vi "FlatToRichgrpc_reflection_v1alpha_ServerReflectionResponse.vi"(5 "OutputClusterType":T1, 11 "InputCluster":T3) -> (3 "OutputCluster":T1)   [LabVIEW 2025, in "reflection_server.lvlib"]
uses:
  reflection_server.lvlib
  grpc_reflection_v1alpha_ServerReflectionResponse_Flat.ctl
  grpc_reflection_v1alpha_ServerReflectionRequest_Flat.ctl
  grpc_reflection_v1alpha_ExtensionRequest_Flat.ctl
  grpc_reflection_v1alpha_FileDescriptorResponse_Flat.ctl
  grpc_reflection_v1alpha_ExtensionNumberResponse_Flat.ctl
  grpc_reflection_v1alpha_ListServiceResponse_Flat.ctl
  grpc_reflection_v1alpha_ServiceResponse_Flat.ctl
  grpc_reflection_v1alpha_ErrorResponse_Flat.ctl
  grpc_reflection_v1alpha_ServerReflectionResponse.ctl
  grpc_reflection_v1alpha_ServerReflectionRequest_message_request/grpc_reflection_v1alpha_ServerReflectionRequest_message_request.lvclass
  grpc_reflection_v1alpha_ServerReflectionResponse_message_response/grpc_reflection_v1alpha_ServerReflectionResponse_message_response.lvclass
  grpc_reflection_v1alpha_ServerReflectionRequest.ctl
  grpc_reflection_v1alpha_ServerReflectionRequest_message_request/grpc_reflection_v1alpha_ServerReflectionRequest_message_request.lvclass/grpc_reflection_v1alpha_ServerReflectionRequest_message_request.ctl
  grpc_reflection_v1alpha_ServerReflectionResponse_message_response/grpc_reflection_v1alpha_ServerReflectionResponse_message_response.lvclass/grpc_reflection_v1alpha_ServerReflectionResponse_message_response.ctl
  grpc_reflection_v1alpha_ServerReflectionRequest_message_request/Setfile_by_filename.vi
  grpc_reflection_v1alpha_ServerReflectionRequest_message_request/Setfile_containing_symbol.vi
  grpc_reflection_v1alpha_ServerReflectionRequest_message_request/Setfile_containing_extension.vi
  FlatToRichgrpc_reflection_v1alpha_ExtensionRequest.vi
  grpc_reflection_v1alpha_ServerReflectionRequest_message_request/Setall_extension_numbers_of_type.vi
  grpc_reflection_v1alpha_ServerReflectionRequest_message_request/Setlist_services.vi
  FlatToRichgrpc_reflection_v1alpha_ServiceResponse.vi
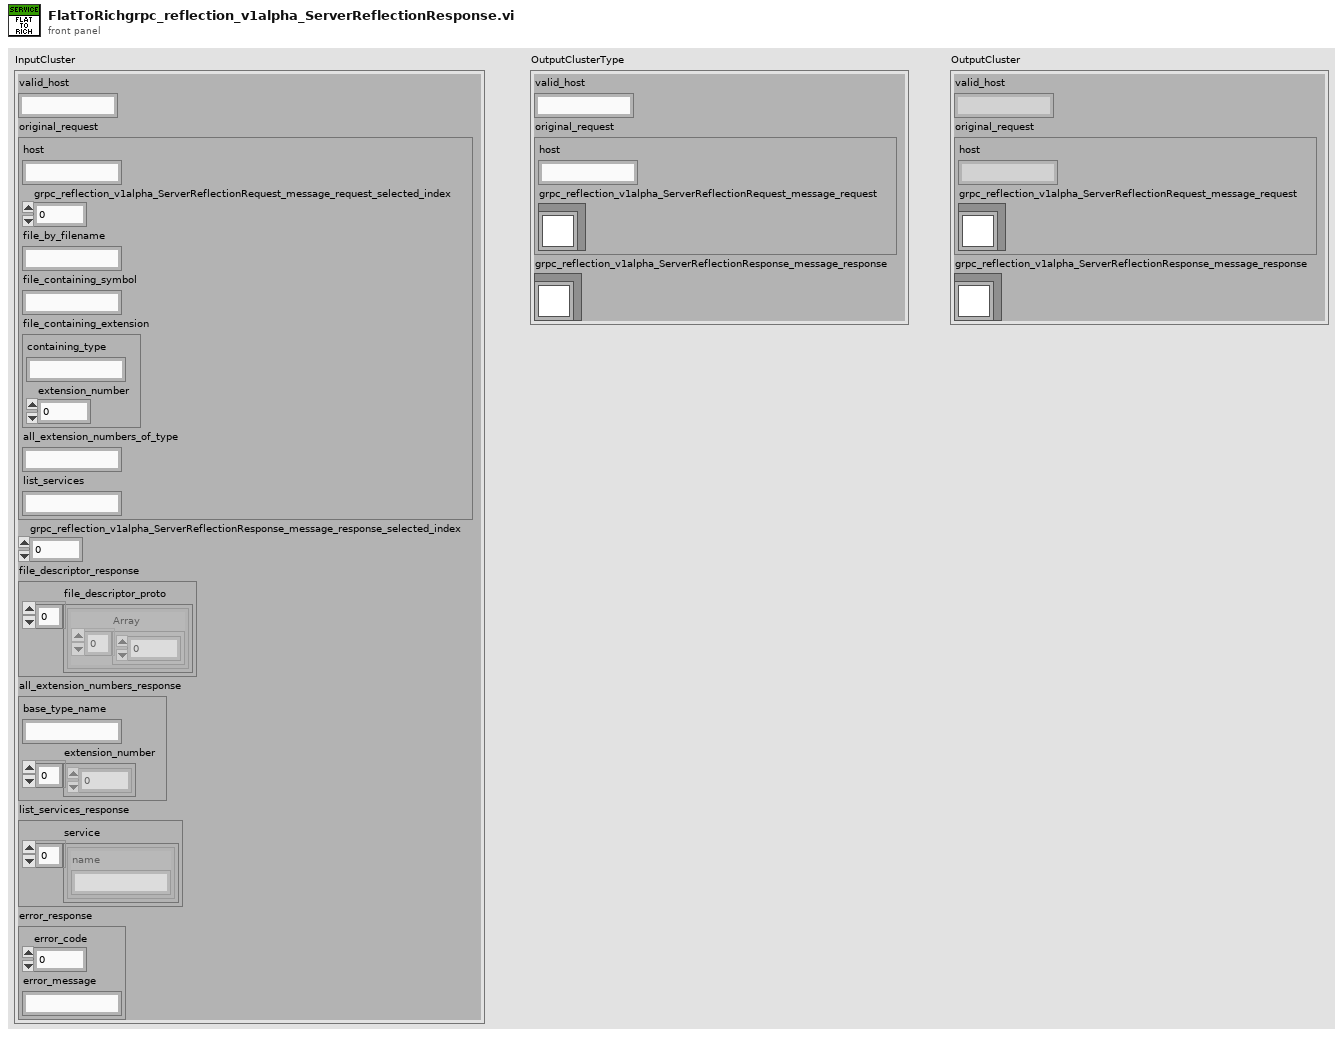
[diagram p1: front panel]
types:
  T1 = typedef "reflection_server.lvlib/grpc_reflection_v1alpha_ServerReflectionResponse.ctl" = cluster{"valid_host":string, "original_request":T2, "grpc_reflection_v1alpha_ServerReflectionResponse_message_response":refnum<class "grpc_reflection_v1alpha_ServerReflectionResponse_message_response.lvclass">}
  T2 = typedef "reflection_server.lvlib/grpc_reflection_v1alpha_ServerReflectionRequest.ctl" = cluster{"host":string, "grpc_reflection_v1alpha_ServerReflectionRequest_message_request":refnum<class "grpc_reflection_v1alpha_ServerReflectionRequest_message_request.lvclass">}
  T3 = typedef "reflection_server.lvlib/grpc_reflection_v1alpha_ServerReflectionResponse_Flat.ctl" = cluster{"valid_host":string, "original_request":T4, "grpc_reflection_v1alpha_ServerReflectionResponse_message_response_selected_index":i32, "file_descriptor_response":T6, "all_extension_numbers_response":T7, "list_services_response":T8, "error_response":T10}
  T4 = typedef "reflection_server.lvlib/grpc_reflection_v1alpha_ServerReflectionRequest_Flat.ctl" = cluster{"host":string, "grpc_reflection_v1alpha_ServerReflectionRequest_message_request_selected_index":i32, "file_by_filename":string, "file_containing_symbol":string, "file_containing_extension":T5, "all_extension_numbers_of_type":string, "list_services":string}
  T5 = typedef "reflection_server.lvlib/grpc_reflection_v1alpha_ExtensionRequest_Flat.ctl" = cluster{"containing_type":string, "extension_number":i32}
  T6 = typedef "reflection_server.lvlib/grpc_reflection_v1alpha_FileDescriptorResponse_Flat.ctl" = cluster{"file_descriptor_proto":cluster{"Array":u8[]}[]}
  T7 = typedef "reflection_server.lvlib/grpc_reflection_v1alpha_ExtensionNumberResponse_Flat.ctl" = cluster{"base_type_name":string, "extension_number":i32[]}
  T8 = typedef "reflection_server.lvlib/grpc_reflection_v1alpha_ListServiceResponse_Flat.ctl" = cluster{"service":T9[]}
  T9 = typedef "reflection_server.lvlib/grpc_reflection_v1alpha_ServiceResponse_Flat.ctl" = cluster{"name":string}
  T10 = typedef "reflection_server.lvlib/grpc_reflection_v1alpha_ErrorResponse_Flat.ctl" = cluster{"error_code":i32, "error_message":string}
  T11 = typedef "reflection_server.lvlib/grpc_reflection_v1alpha_FileDescriptorResponse.ctl" = cluster{"file_descriptor_proto":cluster{"Array":u8[]}[]}
  T12 = typedef "reflection_server.lvlib/grpc_reflection_v1alpha_ExtensionNumberResponse.ctl" = cluster{"base_type_name":string, "extension_number":i32[]}
  T13 = typedef "reflection_server.lvlib/grpc_reflection_v1alpha_ListServiceResponse.ctl" = cluster{"service":T14[]}
  T14 = typedef "reflection_server.lvlib/grpc_reflection_v1alpha_ServiceResponse.ctl" = cluster{"name":string}
  T15 = typedef "reflection_server.lvlib/grpc_reflection_v1alpha_ErrorResponse.ctl" = cluster{"error_code":i32, "error_message":string}
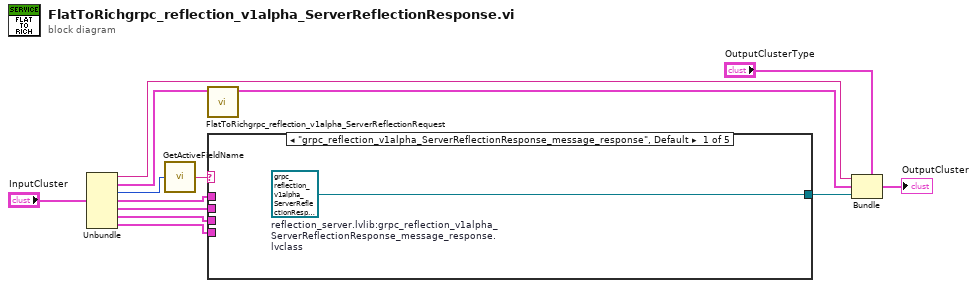
[diagram p0: block diagram]
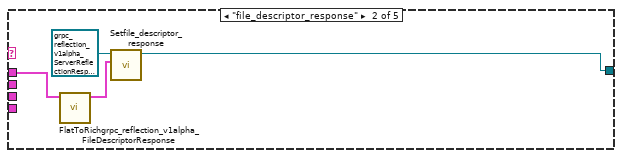
[diagram p2: hidden frame]
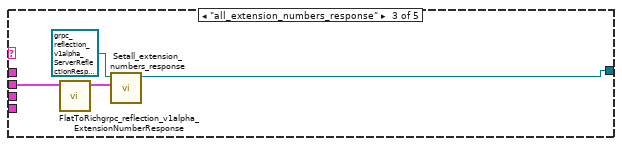
[diagram p3: hidden frame]
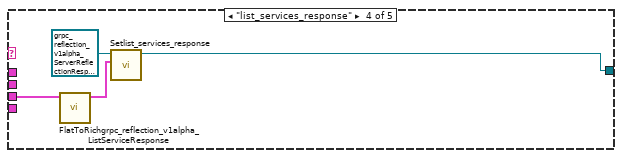
[diagram p4: hidden frame]
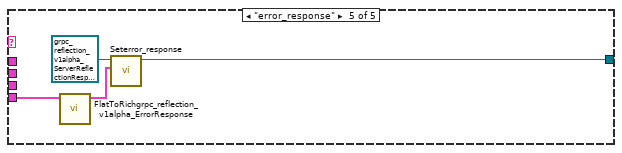
[diagram p5: hidden frame]
diagram:
  n1 = Unbundle "Unbundle"("InputCluster") -> ("valid_host"=w10:string, "original_request"=w9:T4, "grpc_reflection_v1alpha_ServerReflectionResponse_message_response_selected_index"=w7:i32, "file_descriptor_response"=w4:T6, "all_extension_numbers_response"=w3:T7, "list_services_response"=w2:T8, "error_response"=w1:T10)
  n2 = call "GetActiveFieldName.vi"("protobuf index"=w7) -> ("oneof field name"=w6:string)
  n3 = call "FlatToRichgrpc_reflection_v1alpha_ServerReflectionRequest.vi"("InputCluster"=w9) -> ("OutputCluster"=w8:T2)  [unwired: 10 in]
  n4 = case "grpc_reflection_v1alpha_ServerReflectionResponse_message_response" shown="\"grpc_reflection_v1alpha_ServerReflectionResponse_message_response\", Default" w6 {
    tunnel: [w14 w16 w20 w24 w28] -> w5
    tunnel: w4 -> [_ w18 _ _ _]
    tunnel: w3 -> [_ _ w22 _ _]
    tunnel: w2 -> [_ _ _ w26 _]
    tunnel: w1 -> [_ _ _ _ w30]
    frame "grpc_reflection_v1alpha_ServerReflectionResponse_message_response", Default {
      w14 = refnum<class "grpc_reflection_v1alpha_ServerReflectionResponse_message_response.lvclass"> refnum  # reflection_server.lvlib:grpc_reflection_v1alpha_ServerReflectionResponse_message_response.lvclass
    }
    frame "file_descriptor_response" {
      n5 = call "FlatToRichgrpc_reflection_v1alpha_FileDescriptorResponse.vi"("InputCluster"=w18) -> ("OutputCluster"=w17:T11)  [unwired: 10 in]
      n6 = call "Setfile_descriptor_response.vi"("Set_Val"=w17, "OneOfTemplate in"=refnum<class "grpc_reflection_v1alpha_ServerReflectionResponse_message_response.lvclass"> refnum) -> ("OneOfTemplate out"=w16:refnum<class "grpc_reflection_v1alpha_ServerReflectionResponse_message_response.lvclass">)  [unwired: 8 in, 1 out]
    }
    frame "all_extension_numbers_response" {
      n7 = call "FlatToRichgrpc_reflection_v1alpha_ExtensionNumberResponse.vi"("InputCluster"=w22) -> ("OutputCluster"=w21:T12)  [unwired: 10 in]
      n8 = call "Setall_extension_numbers_response.vi"("Set_Val"=w21, "OneOfTemplate in"=refnum<class "grpc_reflection_v1alpha_ServerReflectionResponse_message_response.lvclass"> refnum) -> ("OneOfTemplate out"=w20:refnum<class "grpc_reflection_v1alpha_ServerReflectionResponse_message_response.lvclass">)  [unwired: 8 in, 1 out]
    }
    frame "list_services_response" {
      n9 = call "FlatToRichgrpc_reflection_v1alpha_ListServiceResponse.vi"("InputCluster"=w26) -> ("OutputCluster"=w25:T13)  [unwired: 10 in]
      n10 = call "Setlist_services_response.vi"("Set_Val"=w25, "OneOfTemplate in"=refnum<class "grpc_reflection_v1alpha_ServerReflectionResponse_message_response.lvclass"> refnum) -> ("OneOfTemplate out"=w24:refnum<class "grpc_reflection_v1alpha_ServerReflectionResponse_message_response.lvclass">)  [unwired: 8 in, 1 out]
    }
    frame "error_response" {
      n11 = call "FlatToRichgrpc_reflection_v1alpha_ErrorResponse.vi"("InputCluster"=w30) -> ("OutputCluster"=w29:T15)  [unwired: 10 in]
      n12 = call "Seterror_response.vi"("Set_Val"=w29, "OneOfTemplate in"=refnum<class "grpc_reflection_v1alpha_ServerReflectionResponse_message_response.lvclass"> refnum) -> ("OneOfTemplate out"=w28:refnum<class "grpc_reflection_v1alpha_ServerReflectionResponse_message_response.lvclass">)  [unwired: 8 in, 1 out]
    }
  }
  n13 = Bundle "Bundle"(cluster="OutputClusterType", "valid_host"=w10, "original_request"=w8, "grpc_reflection_v1alpha_ServerReflectionResponse_message_response"=w5) -> (→"OutputCluster":T1)
